vi "FRC Color Connected Components.vi"() -> ()   [LabVIEW 2018]
uses:
  <vilib>/Rock Robotics/SystemInterfaces/spilib/spi_bus.ctl
  source/library/Interface/Pixy Com.lvclass
  source/library/Pixy2.lvlib
  source/deviceSupport/FRC/SPI/RoboRIO SPI.lvclass
panel:
  in  "milliseconds to wait":u32
  in  "signature map":u8=255 format="%.0x"
  in  "max blocks":u8=255
  out "view":picture
  in  "Stop Button":bool
  out "error out":errorcluster
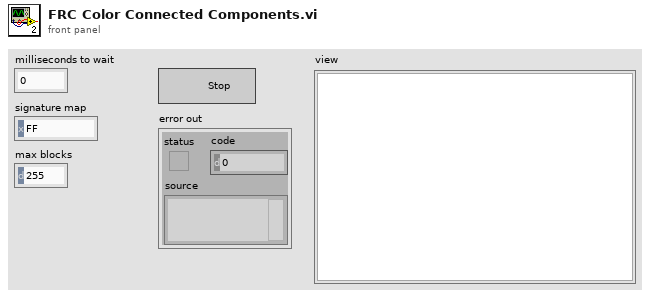
[diagram p1: front panel]
types:
  T1 = typedef "spi_bus.ctl" = enum16{"SPI On-Board, CS0", "SPI On-Board, CS1", "SPI On-Board, CS2", "SPI On-Board, CS3", "SPI MXP", "Invalid"}
  T2 = typedef "Pixy2.lvlib/Block.ctl" = cluster{"signature":u16, "x":u16, "y":u16, "width":u16, "height":u16, "angle":i16, "index":u8, "age":u8}
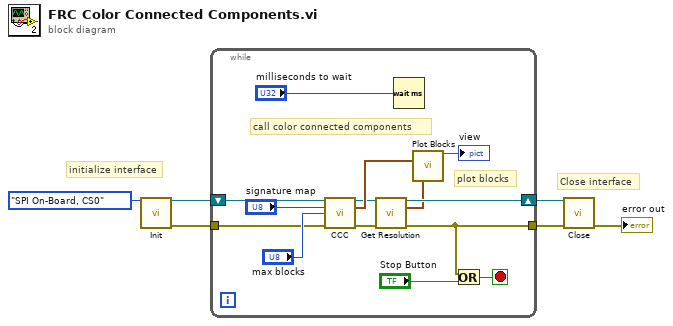
[diagram p0: block diagram]
diagram:
  # "initialize interface"
  # "Close interface"
  n1 = call "Init.vi"("SPI Bus"=spi_bus."SPI On-Board, CS0") -> ("comm interface out"=w6:refnum<class "Pixy Com.lvclass">, "error out"=w1:errorcluster)  [unwired: 13 in]
  n2 = while {
    tunnel: [w18] -> w5
    shift-right: [w19] -> w4
    shift-left: w6 -> [w20]
    tunnel: w1 -> [w7]
    stop <- w17 stop-if-true
    # "plot blocks"
    # "call color connected components"
    n3 = call "CCC.vi"("comm interface in"=w20, "signature map"="signature map", "max blocks"="max blocks", "error in"=w7) -> ("comm interface out"=w11:refnum<class "Pixy Com.lvclass">, "blocks"=w13:T2[], "error out"=w10:errorcluster)  [unwired: 9 in]
    n4 = call "Get Resolution.vi"("comm interface in"=w11, "error in"=w10) -> ("comm interface out"=w19:refnum<class "Pixy Com.lvclass">, "resolution"=w9:cluster{"width":u16, "height":u16}, "error out"=w18:errorcluster)  [unwired: 11 in]
    n5 = Wait (ms)(milliseconds to wait="milliseconds to wait") -> ()  [unwired: 1 out]
    n6 = call "Plot Blocks.vi"("blocks"=w13, "pixy resolution"=w9) -> ("picture out"=→"view":picture)  [unwired: 13 in]
    n7 = Or(x=w18, y="Stop Button") -> (x .or. y?=w17:bool)
  }
  n8 = call-dynamic "Close.vi"("comm interface in"=w4, "error in"=w5) -> ("error out"=→"error out":errorcluster)  [unwired: 13 in]
